vi "Write notifiers.vi"(8 "error in (no error)":errorcluster, 10 "notifier out":refnum<notifier>, 11 "DAQmxTaskContainer in":refnum<class "DAQmxTaskContainer.lvclass">) -> (0 "error out":errorcluster, 3 "DAQmxTaskContainer out":refnum<class "DAQmxTaskContainer.lvclass">)   [LabVIEW 2015, in "DAQmxTaskContainer.lvclass"]
uses:
  DAQmxTaskContainer.lvclass
  DAQmxTaskContainer.lvclass/DAQmxTaskContainer.ctl
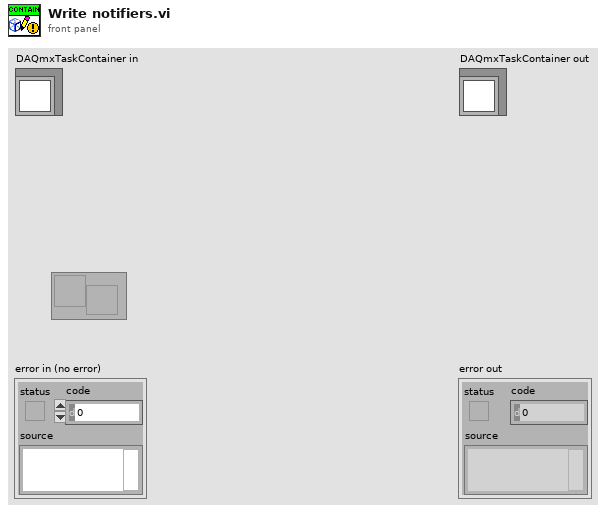
[diagram p1: front panel]
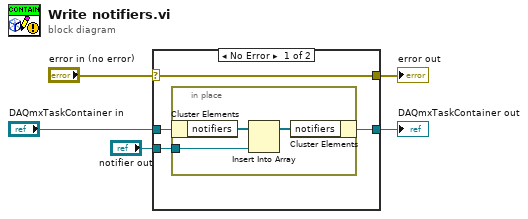
[diagram p0: block diagram]
diagram:
  n1 = case shown="No Error" "error in (no error)" {
    selector: "error in (no error)" -> [w9 w13]
    tunnel: [w9 w13] -> w4
    tunnel: [w7 w14] -> w2
    tunnel: "DAQmxTaskContainer in" -> [w8 w14]
    tunnel: "notifier out" -> [w6 _]
    frame No Error {
      n2 = in-place {
        in-place-border: w6 -> [w10]
        n3 = in-place-cluster #1(w8) -> ("notifiers"=w12:refnum<notifier>[])
        n4 = Insert Into Array(array=w12, new element=w10) -> (w11:refnum<notifier>[])  [unwired: 1 in]
        n5 = in-place-cluster #1("notifiers"=w11) -> (w7:refnum<class "DAQmxTaskContainer.lvclass">)
      }
    }
    frame Error {
    }
  }
  "error out" <- w4
  "DAQmxTaskContainer out" <- w2
